vi "写入固件.vi"(8 "错误输入":errorcluster, 11 "MB session in":refnum<class "MB_Master.lvclass">) -> (0 "error out":errorcluster, 3 "MB session out":refnum<class "MB_Master.lvclass">)   [LabVIEW 2016, in "斯坦道CODMn新电路板.lvlib"]
uses:
  <vilib>/Plasmionique/MB Master/MB_Master/MB_Master.lvclass
  <vilib>/NI/Progress Bar/Controls/Update Bar Actions.ctl
  <vilib>/NI/Progress Bar/Controls/Progress Bar Properties.ctl
  <vilib>/Plasmionique/MB Master/MB_Master_Serial/MB_Master_Serial.lvclass
  D:/Program Files (x86)/National Instruments/LabVIEW 2016/vi.lib/Plasmionique/MB Master/MB_Master/MB_Master.lvclass
  <vilib>/Plasmionique/MB Master/MB Master.lvlib
  <vilib>/NI/Progress Bar/Progress Bar.lvlib
panel:
  in  "引用选择":enum16{"MB引用", "自建引用"}(ring)
  in  "VISA Resource":refnum<visa-resource-name>
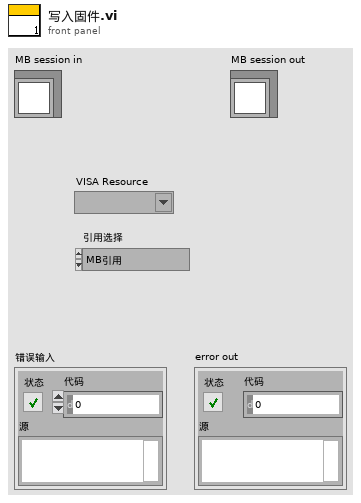
[diagram p1: front panel]
types:
  T1 = enum16{"open", "replace", "create", "open or create", "replace or create", "replace or create with confirmation"}
  T2 = enum16{"big-endian, network order", "native, host order", "little-endian"}
  T3 = typedef "Progress Bar.lvlib/Update Bar Actions.ctl" = enum16{"Add To Existing", "Set to Value"}
  T4 = cluster{"baud rate (bps)":u32, "stop bits":u16, "parity":u16, "flow control":u16, "timeout":u32, "retries":i32}
  T5 = typedef "Progress Bar.lvlib/Progress Bar Properties.ctl" = cluster{"Background Color":u32, "Installer Title":string, "Title Color":u32, "Action Text":string, "Text Color":u32, "Slider Value":u8, "Bar Color":u32, "Timeout":i32}
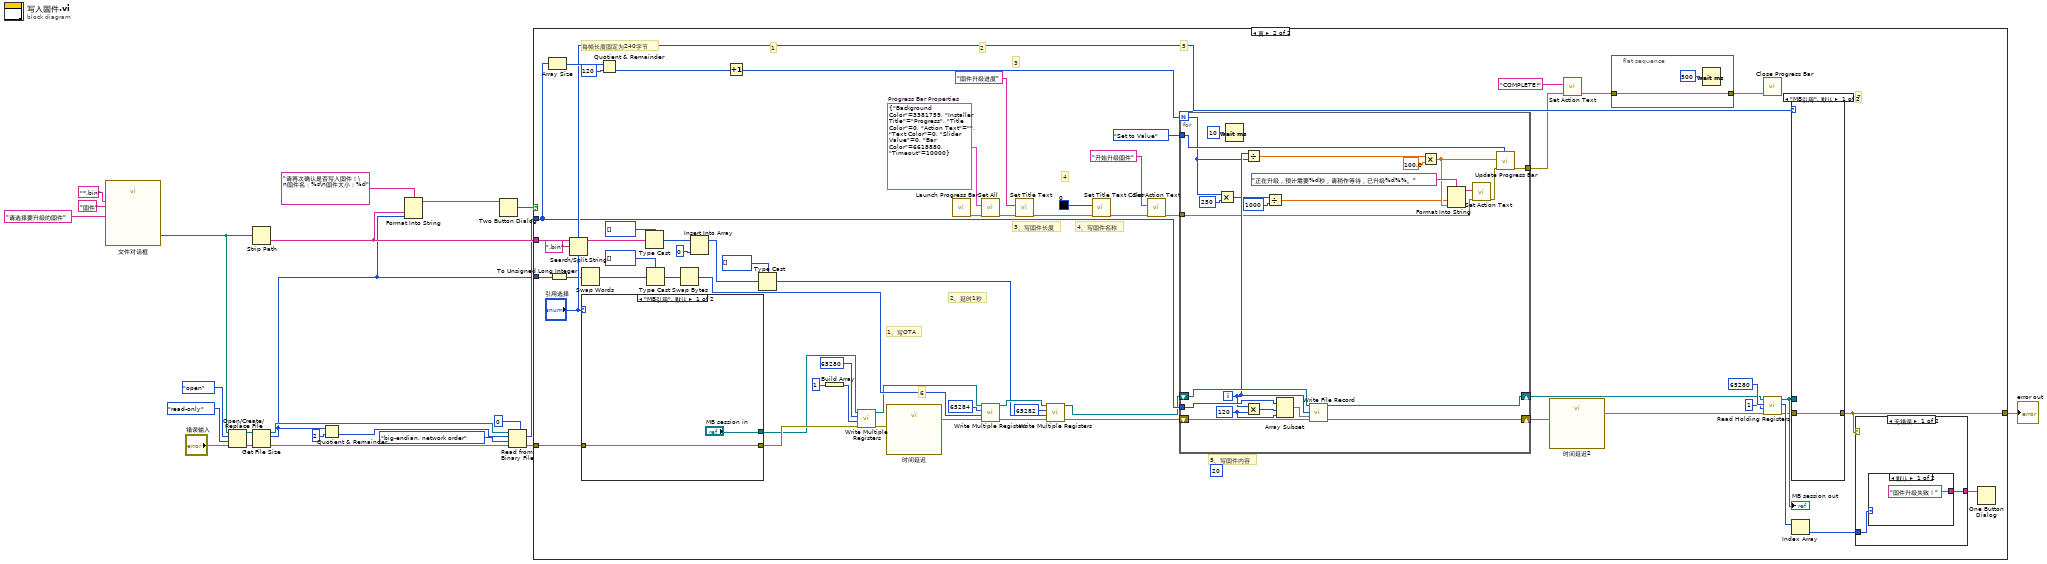
[diagram p0: block diagram]
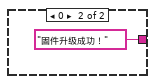
[diagram p3: hidden frame]
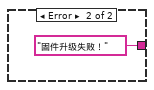
[diagram p4: hidden frame]
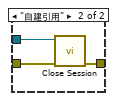
[diagram p5: hidden frame]
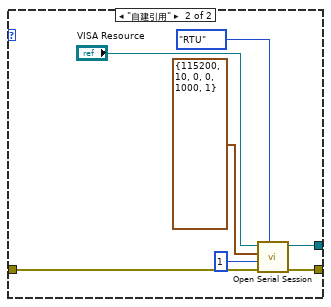
[diagram p6: hidden frame]
diagram:
  n1 = call "文件对话框"("prompt"="请选择要升级的固件", "pattern (all files)"="*.bin", "pattern label"="固件") -> ("selected path"=w10:path)  [unwired: 9 in, 3 out]
  n2 = Open/Create/Replace File(file path (use dialog)=w10, error in="错误输入", operation (0:open)=T1."open" ("操作(0:open)"), access (0:read/write)=enum16{"read/write", "read-only", "write-only"}."read-only" ("权限(0:read/write)")) -> (refnum out=w9:refnum<file>, error out=w7:errorcluster)  [unwired: 2 in, 1 out]
  n3 = Strip Path(path=w10) -> (name=w18:string)  [unwired: 1 out]
  n4 = Get File Size(file=w9, error in=w7) -> (refnum out=w8:refnum<file>, size (in bytes)=w2:i64, 0:w6:errorcluster)
  n5 = Quotient & Remainder(x=w2, y=i64 2) -> (floor(x/y)=w4:i64)  [unwired: 1 out]
  n6 = Format Into String(format string="请再次确认是否写入固件！\n固件名：%s\n固件大小：%d" ("格式字符串"), w18, w2) -> (resulting string=w17:string)  [unwired: 2 in, 1 out]
  n7 = Two Button Dialog(message=w17) -> (T button?=w16:bool)  [unwired: 2 in]
  n8 = Read from Binary File(5:u16 0, 8:w6, 9:T2."big-endian, network order" ("字节顺序(0:big-endian, network order)"), 10:w4, 11:w8) -> (0:w15:errorcluster, 2:w3:u16[])  [unwired: 1 in, 2 out]
  n9 = case shown="真" w16 {
    tunnel: w3 -> [_ w51]
    tunnel: w18 -> [_ w67]
    tunnel: w15 -> [w24 w69]
    tunnel: [w24 w47] -> w13
    tunnel: w2 -> [_ w53]
    frame False {
    }
    frame True {
      w44 = T5 {"Background Color"=3381759, "Installer Title"="Progress", "Title Color"=0, "Action Text"="", "Text Color"=0, "Slider Value"=0, "Bar Color"=6618880, "Timeout"=10000}  # Progress Bar Properties
      (unwired) 20 ("Value")
      # "7"
      # "6"
      # "5"
      # "4"
      # "3"
      # "2"
      # "1"
      # "每帧长度固定为240字节"
      # "5、写固件内容"
      # "4、写固件名称"
      # "3、写固件长度"
      # "2、延时1秒"
      # "1、写OTA"
      n10 = Array Size(array=w51) -> (size(s)=w84:i32)
      n11 = To Unsigned Long Integer(number=w53) -> (unsigned 32bit integer=w50:u32)
      n12 = Search/Split String(string=w67, search string/char (-)=".bin" ("搜索字符串/字符(-)")) -> (substring before match=w65:string)  [unwired: 1 in, 2 out]
      n13 = Swap Words(1:w50) -> (0:w49:u32)
      n14 = case shown="\"MB引用\", 默认" "引用选择" {
        tunnel: ["MB session in" w104] -> w25
        tunnel: w69 -> [w98 w103]
        tunnel: [w98 w102] -> w30
        frame "MB引用", Default {
        }
        frame "自建引用" {
          n15 = call <vilib>:"Open Serial Session.vi"("Mode (RTU)"=enum16{"RTU", "ASCII"}."RTU", "Error in"=w103, "Slave ID"=u8 1, "Serial Config"=T4 {"baud rate (bps)"=115200, "stop bits"=10, "parity"=0, "flow control"=0, "timeout"=1000, "retries"=1}, "VISA Resource"="VISA Resource") -> ("Error out"=w102:errorcluster, "MB_Serial session"=w104:refnum<class "MB_Master_Serial.lvclass">)  [unwired: 5 in]
        }
      }
      n16 = Quotient & Remainder(x=w84, y=120) -> (floor(x/y)=w85:i32)  [unwired: 1 out]
      n17 = Type Cast(type=u8[] [], x=w65) -> (*(type *) &x=w72:u8[])
      n18 = Type Cast(type=u16[] [], x=w49) -> (*(type *) &x=w78:u16[])
      n19 = Swap Bytes(anything=w78) -> (byte swapped=w77:u16[])
      n20 = Insert Into Array(array=w72, new element=u8 0 ("新元素/子数组")) -> (w64:u8[])  [unwired: 1 in]
      n21 = Increment(x=w85) -> (x+1=w52:i32)
      n22 = Type Cast(type=u16[] [], x=w64) -> (*(type *) &x=w63:u16[])
      n23 = Build Array(u16 1 ("value")) -> (w70:u16[])
      n24 = call <vilib>:"Write Multiple Registers.vi"("error in (no error)"=w30, "values"=w70, "starting address"=u16 65280, "MB session in"=w25) -> ("error out"=w80:errorcluster, "MB session out"=w56:refnum<class "MB_Master.lvclass">)  [unwired: 6 in]
      n25 = call "时间延迟"("error in (no error)"=w80) -> ("error out"=w57:errorcluster)  [unwired: 10 in]
      n26 = call <vilib>:"Launch Progress Bar.vi"() -> ("error out"=w43:errorcluster)  [unwired: 10 in, 1 out]
      n27 = call <vilib>:"Set All.vi"("error in (no error)"=w43, "Progress Bar Properties (Default)"=w44) -> ("error out"=w37:errorcluster)  [unwired: 9 in]
      n28 = call <vilib>:"Write Multiple Registers.vi"("error in (no error)"=w57, "values"=w77, "starting address"=u16 65284, "MB session in"=w56) -> ("error out"=w75:errorcluster, "MB session out"=w76:refnum<class "MB_Master.lvclass">)  [unwired: 6 in]
      n29 = call <vilib>:"Set Title Text.vi"("error in (no error)"=w37, "Installer Title"="固件升级进度") -> ("error out"=w35:errorcluster)  [unwired: 9 in]
      n30 = call <vilib>:"Write Multiple Registers.vi"("error in (no error)"=w75, "values"=w63, "starting address"=u16 65282, "MB session in"=w76) -> ("error out"=w28:errorcluster, "MB session out"=w29:refnum<class "MB_Master.lvclass">)  [unwired: 6 in]
      n31 = call <vilib>:"Set Title Text Color.vi"("error in (no error)"=w35, "Color Box"=u32 0) -> ("error out"=w38:errorcluster)  [unwired: 9 in]
      n32 = call <vilib>:"Set Action Text.vi"("error in (no error)"=w38, "Action Text"="开始升级固件") -> ("error out"=w32:errorcluster)  [unwired: 9 in]
      n33 = for {
        N: w52 -> [w107]
        shift-right: [w127] -> w26
        shift-left: w29 -> [w129]
        shift-right: [w125] -> w48
        shift-left: w28 -> [w128]
        tunnel: w51 -> [w124]
        tunnel: Update_Bar_Actions."Set to Value" ("Action") -> [w119]
        tunnel: w32 -> [w117]
        tunnel: [w118] -> w31
        i -> [w122]
        w121 = 120 ("长度")
        n34 = Multiply(x=w107, y=250) -> (x*y=w111:i32)
        n35 = Wait (ms)(milliseconds to wait=u32 10) -> ()  [unwired: 1 out]
        n36 = Divide(x=w122, y=w107) -> (x/y=w113:dbl)
        n37 = Multiply(x=w122, y=w121) -> (x*y=w120:i32)
        n38 = Divide(x=w111, y=u32 1000) -> (x/y=w108:dbl)
        n39 = Array Subset(array=w124, index=w120, length=w121) -> (w123:u16[])
        n40 = call "Write File Record.vi"("MB session in"=w129, "Record Number"=w122, "values"=w123, "error in (no error)"=w128) -> ("MB session out"=w127:refnum<class "MB_Master.lvclass">, "error out"=w125:errorcluster)  [unwired: 10 in]
        n41 = Multiply(x=w113, y=100.0) -> (x*y=w109:dbl)
        n42 = Format Into String(format string="正在升级，预计需要%d秒，请稍作等待，已升级%d%%。" ("格式字符串"), w108, w109) -> (resulting string=w114:string)  [unwired: 2 in, 1 out]
        n43 = call <vilib>:"Set Action Text.vi"("error in (no error)"=w117, "Action Text"=w114) -> ("error out"=w116:errorcluster)  [unwired: 9 in]
        n44 = call <vilib>:"Update Progress Bar.vi"("Action"=w119, "error in (no error)"=w116, "Value"=w109) -> ("error out"=w118:errorcluster)  [unwired: 8 in]
      }
      n45 = call "时间延迟2"("error in (no error)"=w48) -> ("error out"=w27:errorcluster)  [unwired: 10 in]
      n46 = call <vilib>:"Set Action Text.vi"("error in (no error)"=w31, "Action Text"="COMPLETE!") -> ("error out"=w40:errorcluster)  [unwired: 9 in]
      n47 = flat-sequence {
        tunnel: w40 -> [w86]
        tunnel: [w86] -> w42
        frame #0 {
          n48 = Wait (ms)(milliseconds to wait=u32 500) -> ()  [unwired: 1 out]
        }
      }
      n49 = call <vilib>:"Close Progress Bar.vi"("error in (no error)"=w42) -> ()  [unwired: 9 in, 2 out]
      n50 = call <vilib>:"Read Holding Registers.vi"("error in (no error)"=w27, "quantity"=u16 1, "starting address"=u16 65280, "MB session in"=w26) -> ("error out"=w54:errorcluster, "Registers"=w58:u16[], "MB session out"=w55:refnum<class "MB_Master.lvclass">)  [unwired: 5 in]
      "MB session out" <- w55
      n51 = case shown="\"MB引用\", 默认" "引用选择" {
        tunnel: w55 -> [_ w96]
        tunnel: w54 -> [w93 w95]
        tunnel: [w93 w94] -> w47
        frame "MB引用", Default {
        }
        frame "自建引用" {
          n52 = call-dynamic "Close Session.vi"("error in (no error)"=w95, "MB session in"=w96) -> ("error out"=w94:errorcluster)  [unwired: 9 in]
        }
      }
      n53 = Index Array(array=w58) -> (element=w46:u16)  [unwired: 1 in]
      n54 = case shown="无错误" w47 {
        tunnel: w46 -> [w89 _]
        tunnel: [w88 "固件升级失败！"] -> w45
        frame No Error {
          n55 = case shown="默认" w89 {
            tunnel: ["固件升级失败！" "固件升级成功！"] -> w88
            frame Default {
            }
            frame 0 {
            }
          }
        }
        frame Error {
        }
      }
      n56 = One Button Dialog(message=w45) -> ()  [unwired: 1 in, 1 out]
    }
  }
  "error out" <- w13
